vi "niFpgaPID_PIDMemoryWrite.vi"(0 "memory in":refnum<k21>="Data", 1 "channel (0)":u8, 11 "state in":T2, 12 "parameters in":T1) -> ()   [LabVIEW 2017]
uses:
  <vilib>/rvi/Analysis/control/PID/Typedef/niFpgaPID_PIDState.ctl
  <vilib>/rvi/Analysis/control/PID/Typedef/niFpgaPID_PIDParameters.ctl
  <vilib>/rvi/Analysis/control/PID/Typedef/niFpgaPID_PIDMemoryItem.ctl
  <vilib>/Platform/TimedLoop/XDataNode/timing_clust.ctl
  <vilib>/Platform/TimedLoop/XDataNode/nitl_modes.ctl
  <vilib>/Platform/TimedLoop/XDataNode/wakeup.ctl
  <vilib>/rvi/Emulation/niFpgaSctlEmulationGetInTimedLoop.vi
  <vilib>/Utility/error.llb/Clear Errors.vi
  <vilib>/rvi/DataTransferAndStorage/Container/Common/niFpgaContainerExecOnDevCompGetState.vi
  <vilib>/rvi/Emulation/niFpgaEmulationIsFPGAContextNoSignature.vi
  <vilib>/rvi/DataTransferAndStorage/Container/Common/niFpgaContainerGetUniqueNameForEmu.vi
  <vilib>/rvi/Emulation/niFpgaProcessEmulError.vi
  <vilib>/rvi/errors/nirviReportUnexpectedCaseInternalError (U32).vi
  <vilib>/rvi/Memory/Memory_Emulation/niFpgaMemoryEmulationCacheClearOnFirstRun.vi
  <vilib>/rvi/Memory/Memory_Emulation/nirvimemoryEmulationManagerCache_MakeExclusive.vi
  <vilib>/rvi/Memory/Memory_Emulation/niFpgaMemoryEmulationValidateCache.vi
  <vilib>/rvi/Memory/Memory_Emulation/nirvimemoryEmulationManagerCache_InsertValue.vi
  <vilib>/rvi/Memory/Memory_Emulation/nirvimemoryEmulationManagerCache_ReleaseExclusive.vi
  <vilib>/rvi/Memory/Memory_Emulation/nirvimemoryEmulationManagerCache_GetValue.vi
  <vilib>/rvi/Memory/Memory_Emulation/nirvimemoryEmulationManagerCache_SetValue.vi
  <vilib>/rvi/Emulation/niFpgaSctlEmulationResourceMgr.vi
  <vilib>/Platform/TimedLoop/XDataNode/XDataNode.xnode
  <vilib>/rvi/DataTransferAndStorage/Container/XNode/niFpgaContainer.xnode
  <vilib>/rvi/Memory/Memory_Emulation/niFpgaMemoryEmulationRefIn.vi
  <vilib>/Platform/TimedLoop/XDataNode/XDNodeRunTimeDep.lvlib
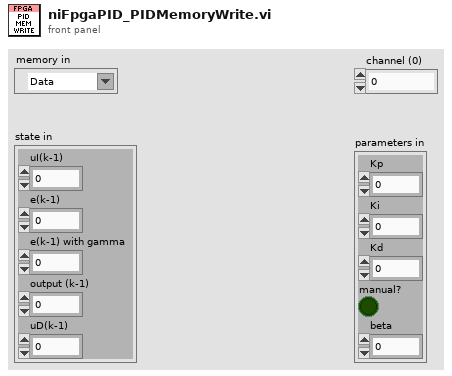
[diagram p1: front panel]
types:
  T1 = typedef "niFpgaPID_PIDParameters.ctl" = cluster{"Kp":sgl, "Ki":sgl, "Kd":sgl, "manual?":bool, "beta":sgl}
  T2 = typedef "niFpgaPID_PIDState.ctl" = cluster{"uI(k-1)":sgl, "e(k-1)":sgl, "e(k-1) with gamma":sgl, "output (k-1)":sgl, "uD(k-1)":sgl}
  T3 = typedef "niFpgaPID_PIDMemoryItem.ctl" = cluster{"data 1":sgl, "data 2":sgl, "data 3":sgl, "data 4":sgl, "data 5":sgl}
  T4 = typedef "XDNodeRunTimeDep.lvlib/timing_clust.ctl" = cluster{"Expected End [f-1]":u64, "Actual End [f-1]":u64, "Finished Late? [f-1]":bool, "Expected End [i-1]":u64, "Actual End [i-1]":u64, "Finished Late? [i-1]":bool, "Expected Start [i]":u64, "Actual Start [i]":u64, "Expected Start [f]":u64, "Actual Start [f]":u64, "Source Name":string, "Structure Name":string, "Period":i64, "Deadline":i64, "Offset":i64, "Start":i64, "Priority":i32, "Timeout":i32, "Mode":T5, "Wakeup Reason":T6, "Error":errorcluster, "Source Type":string, "Secondary Source Type":string, "Global End Time":u64, "Global Start Time":u64, "Frame Duration":u64, "Iteration Duration":u64, "Assigned CPU":i32, "I/O Scan Engine Mode":u32}
  T5 = typedef "XDNodeRunTimeDep.lvlib/nitl_modes.ctl" = enum32{"No Change", "Process missed periods, maintain original phase", "Discard missed periods, maintain original phase", "Process missed periods, ignore original phase", "Discard missed periods, ignore original phase"}
  T6 = typedef "XDNodeRunTimeDep.lvlib/wakeup.ctl" = enum32{"Normal", "Aborted", "Asynchronous wakeup", "Timing source error", "Timed loop error", "Timeout"}
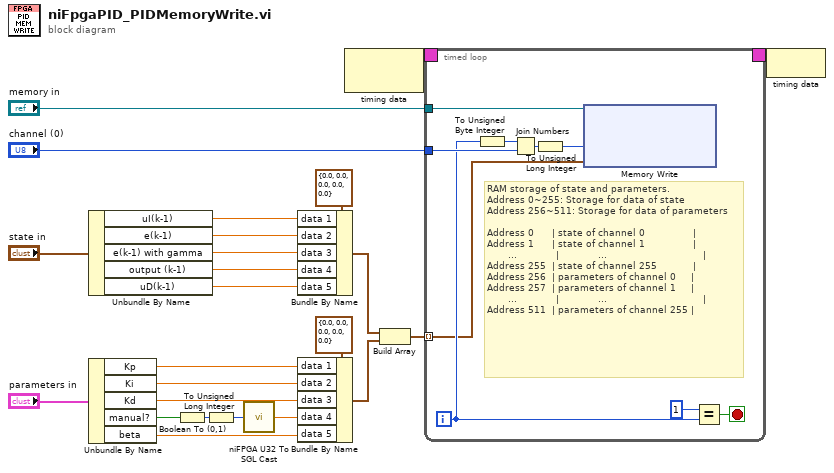
[diagram p0: block diagram]
diagram:
  n1 = Unbundle By Name("state in") -> ("uI(k-1)"=w13:sgl, "e(k-1)"=w9:sgl, "e(k-1) with gamma"=w10:sgl, "output (k-1)"=w11:sgl, "uD(k-1)"=w12:sgl)
  n2 = Unbundle By Name("parameters in") -> ("Kp"=w8:sgl, "Ki"=w7:sgl, "Kd"=w6:sgl, "manual?"=w2:bool, "beta"=w5:sgl)
  n3 = Boolean To (0,1)(Boolean=w2) -> (0, 1=w19:i16)
  n4 = To Unsigned Long Integer(number=w19) -> (unsigned 32bit integer=w4:u32)
  n5 = call <vilib>:"niFPGA U32 To SGL Cast.vi"("x"=w4) -> ("y"=w3:sgl)  [unwired: 4 in]
  n6 = Bundle By Name(cluster=T3 {"data 1"=0.0, "data 2"=0.0, "data 3"=0.0, "data 4"=0.0, "data 5"=0.0} ("PID memory dummy type"), "data 1"=w13, "data 2"=w9, "data 3"=w10, "data 4"=w11, "data 5"=w12) -> (w16:T3)
  n7 = Bundle By Name(cluster=T3 {"data 1"=0.0, "data 2"=0.0, "data 3"=0.0, "data 4"=0.0, "data 5"=0.0} ("PID memory dummy type"), "data 1"=w8, "data 2"=w7, "data 3"=w6, "data 4"=w3, "data 5"=w5) -> (w15:T3)
  n8 = node-c288() -> (w24:T4)  [unwired: 1 in]
  n9 = Build Array(w16, w15) -> (w14:T3[])
  n10 = timed-loop {
    timing: w24 -> [_]
    timing-out: [_] -> w23
    tunnel: "memory in" -> [w33]
    tunnel: "channel (0)" -> [w30]
    tunnel: w14 -> [w25] mode=indexing
    i -> [w28]
    stop <- w32 stop-if-true
    # "RAM storage of state and parameters. \nAddress 0~255: Storage for data of state\nAddress 256~511: Storage for data of parameters\n                                                                         \nAddress 0      | state of channel 0                | \nAddress 1      | state of channel 1                | \n       ...             |             ...                                |\nAddress 255  | state of channel 255            | \nAddress 256  | parameters of channel 0     | \nAddress 257  | parameters of channel 1     | \n       ...             |             ...                                |\nAddress 511  | parameters of channel 255 |"
    n11 = To Unsigned Byte Integer(number=w28) -> (unsigned 8bit integer=w27:u8)
    n12 = Join Numbers(hi=w27, lo=w30) -> ((hi.lo)=w31:u16)
    n13 = To Unsigned Long Integer(number=w31) -> (unsigned 32bit integer=w29:u32)
    n14 = xnode "Memory Write"("Address"=w29, "Data"=w25, "Memory In"=w33) -> ()  [unwired: 1 out]
    n15 = Equal?(x=1, y=w28) -> (x = y?=w32:bool)
  }
  n16 = node-c288(w23) -> ()
